vi "Convert SequenceFile Type.vi"(10 "SequenceFile Type":T1, 11 "TS API":i32(ring) items=["SeqFileType_Normal", "SeqFileType_Model", "SeqFileType_FrontEndCBacks", "SeqFileType_StationCBacks", "SeqFileType_Template"]) -> (2 "TSnax -> TS API":i32(ring) items=["SeqFileType_Normal", "SeqFileType_Model", "SeqFileType_FrontEndCBacks", "SeqFileType_StationCBacks", "SeqFileType_Template"], 3 "TS API -> TSnax":T1)   [LabVIEW 2020, in "TSnax.lvlib"]
uses:
  TSnax.lvlib
  SequenceFile Type.ctl
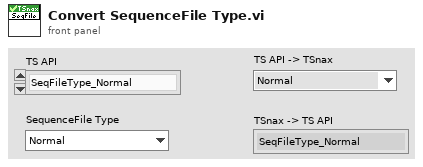
[diagram p1: front panel]
types:
  T1 = typedef "TSnax.lvlib/SequenceFile Type.ctl" = enum16{"Normal", "Model", "Front End Callbacks", "Station Callbacks", "Template"}
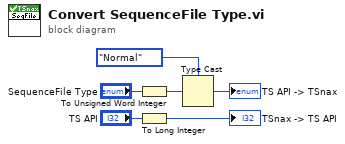
[diagram p0: block diagram]
diagram:
  n1 = To Unsigned Word Integer(number="SequenceFile Type") -> (unsigned 16bit integer=w5:u16)
  n2 = To Long Integer(number="TS API") -> (32bit integer=→"TSnax -> TS API":i32)
  n3 = Type Cast(type=SequenceFile_Type."Normal" ("TS API -> TSnax"), x=w5) -> (*(type *) &x=→"TS API -> TSnax":T1)
